vi "Request Timed Out--error.vi"(10 "Module ID":i32=-1, 11 "Request":string) -> (0 "error out":errorcluster)   [LabVIEW 2020, in "GenNet-Client.lvlib"]
doc: "Outputs an error cluster containing a custom error code indicating a request and wait for reply timed out.\n____\nHAMPEL SOFTWARE ENGINEERING v3.8.0 (2023-12-18 14:41)"
uses:
  GenNet-Client.lvlib
  <vilib>/Utility/error.llb/Error Cluster From Error Code.vi
  <vilib>/ErrorRing/Error Ring.xnode
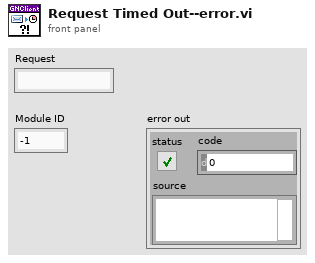
[diagram p1: front panel]
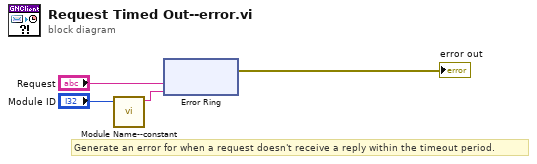
[diagram p0: block diagram]
diagram:
  # "Generate an error for when a request doesn't receive a reply within the timeout period."
  n1 = call "Module Name--constant.vi"("Module ID"="Module ID") -> ("Module Name"=w3:string)  [unwired: 10 in]
  n2 = xnode "Error Ring"("parameter 0"="Request", "parameter 1"=w3) -> ("error out"=→"error out":errorcluster)
